vi "Optimization.vi"() -> ()   [LabVIEW 2020]
uses:
  <vilib>/MakerHub/LINX/Public/Peripherals/Digital/Digital Read 1 Chan.vi
  <vilib>/MakerHub/LINX/Public/Peripherals/PWM/PWM Set Duty Cycle 1 Chan.vi
  <vilib>/MakerHub/LINX/Public/Peripherals/Digital/Digital Read N Chans.vi
  <vilib>/MakerHub/LINX/Private/Local IO/LinxDigitalRead.vi
  <vilib>/MakerHub/LINX/Public/Utilities/Check Channel.vi
  <vilib>/MakerHub/LINX/Public/Utilities/Open Serial.vi
  <vilib>/MakerHub/LINX/Private/Utilties/Generate Error.vi
  <vilib>/MakerHub/LINX/Public/Peripherals/PWM/PWM Set Duty Cycle N Chans.vi
  <vilib>/MakerHub/LINX/LMH-LINX.lvlib
panel:
  out "Thermometer":dbl(slide) scale=0.0..100.0
  out "Light intensity":dbl
  out "Temperature":dbl
  out "Motion detection":bool
  out "Fan speed level":dbl
  out "Wind speed":dbl
  in  "stop":bool
  in  "Serial Port":refnum<visa-resource-name>="N/A"
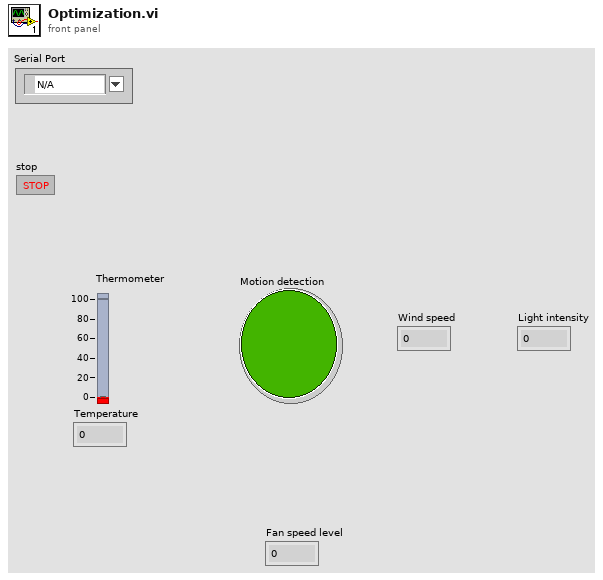
[diagram p1: front panel]
types:
  T1 = typedef "LMH-LINX.lvlib/LINX Ref.ctl" = cluster{"IO":T2, "Interface":T3, "LINX Device Config":T4}
  T2 = typedef "LMH-LINX.lvlib/Platform.ctl" = enum16{"Remote", "Local"}
  T3 = typedef "LMH-LINX.lvlib/Interface.ctl" = enum16{"Serial", "TCP"}
  T4 = typedef "LMH-LINX.lvlib/Device.lvlib/LINX Device Config.ctl" = cluster{"Interface":T3, "COM Port":refnum<visa-resource-name>, "TCP Configuration":T5, "Device Family":u8, "Device ID":u8, "Device Name":string, "TCP Ref":refnum<k5>, "Channels":T6}
  T5 = typedef "LMH-LINX.lvlib/Device.lvlib/TCP Config.ctl" = cluster{"IP Address":string, "Port":u16}
  T6 = typedef "LMH-LINX.lvlib/Channels.ctl" = cluster{"DI":u8[], "DO":u8[], "AI":u8[], "AO":u8[], "PWM":u8[], "QE":u8[], "UART":u8[], "I2C 2":u8[], "SPI":u8[], "CAN":u8[], "Servo":u8[], "AI Ref (V)":dbl, "AI Resolution (Bits)":u8, "AO Ref (V)":dbl, "AO Resolution (Bits)":u8}
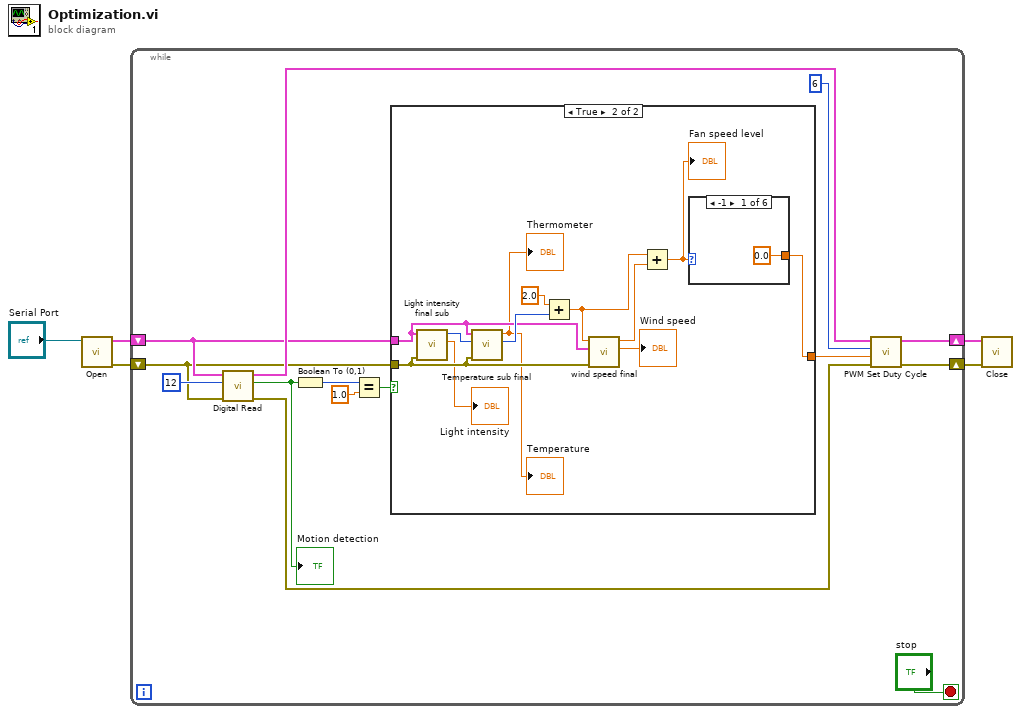
[diagram p0: block diagram]
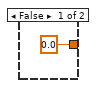
[diagram p2: hidden frame]
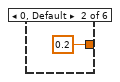
[diagram p3: hidden frame]
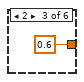
[diagram p4: hidden frame]
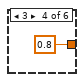
[diagram p5: hidden frame]
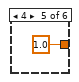
[diagram p6: hidden frame]
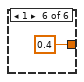
[diagram p7: hidden frame]
diagram:
  n1 = call-poly <vilib>:"Open.vi"("Serial Port"="Serial Port") -> ("Error Out"=w2:errorcluster, "LINX Resource"=w4:T1)  [unwired: 8 in, 1 out]
  n2 = while {
    shift-right: [w18] -> w3
    shift-left: w4 -> [w10]
    shift-right: [w16] -> w1
    shift-left: w2 -> [w9]
    stop <- "stop" stop-if-true
    n3 = call-poly <vilib>:"Digital Read.vi"("Error In"=w9, "DI Channel"=u8 12, "LINX Resource"=w10) -> ("Error Out"=w8:errorcluster, "DI Value"=w15:bool, "LINX Resource"=w11:T1)  [unwired: 6 in]
    "Motion detection" <- w15
    n4 = Boolean To (0,1)(Boolean=w15) -> (0, 1=w13:i16)
    n5 = Equal?(x=w13, y=1.0) -> (x = y?=w6:bool)
    n6 = case shown="True" w6 {
      tunnel: w10 -> [_ w26]
      tunnel: w9 -> [_ w25]
      tunnel: [0.0 w32] -> w7
      frame False {
      }
      frame True {
        n7 = call "Light intensity final sub.vi"("error in (no error)"=w25, "LINX Resource"=w26) -> ("Voltage"=→"Light intensity":dbl, "Numeric"=w31:i32)  [unwired: 8 in]
        n8 = call "Temperature sub final.vi"("error in (no error)"=w25, "Numeric 3"=w31, "LINX Resource"=w26) -> ("Numeric 2"=w29:i32, "Numeric"=→"Temperature" →"Thermometer":dbl)  [unwired: 7 in]
        n9 = Add(x=2.0, y=w29) -> (x+y=w24:dbl)
        n10 = call "wind speed final.vi"("error in (no error)"=w25, "LINX Resource"=w26, "Numeric 3"=w24) -> ("Numeric 2"=→"Wind speed":dbl, "Numeric 4"=w27:dbl)  [unwired: 7 in]
        n11 = Add(x=w24, y=w27) -> (x+y=w28:dbl)
        "Fan speed level" <- w28
        n12 = case shown="-1" w28 {
          tunnel: [0.0 0.2 0.6 0.8 1.0 0.4] -> w32
          frame -1 {
          }
          frame 0, Default {
          }
          frame 2 {
          }
          frame 3 {
          }
          frame 4 {
          }
          frame 1 {
          }
        }
      }
    }
    n13 = call-poly <vilib>:"PWM Set Duty Cycle.vi"("Error In"=w8, "Duty Cycle (0-1)"=w7, "PWM Channel"=u8 6, "LINX Resource"=w11) -> ("Error Out"=w16:errorcluster, "LINX Resource"=w18:T1)  [unwired: 6 in]
  }
  n14 = call <vilib>:"Close.vi"("Error In"=w1, "LINX Resource"=w3) -> ()  [unwired: 9 in, 1 out]
